vi "Helper - overlay optimal heading.vi"(6 "Line length (px)":dbl=500.0, 8 "Overlay Color":u32(colorbox)=6618880, 9 "Boat Image Coords":cluster{"X":i32, "Y":i32}, 10 "Optimal Heading":T2 format="%05.1f", 11 "Image In":T1) -> (3 "Image Out":T1)   [LabVIEW 2011]
doc: "overlays a line indicating the direction that the boat 'wants' to go.\nby Jason Curtis"
uses:
  <vilib>/vision/Image Controls.llb/IMAQ Image.ctl
  2-Think/2 Typedefs/heading.ctl
panel:
  out "Start Point":cluster{"X":i32, "Y":i32}
  out "End Point":cluster{"X":i32, "Y":i32}
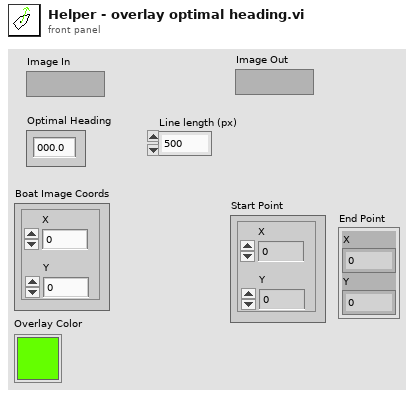
[diagram p1: front panel]
types:
  T1 = typedef "IMAQ Image.ctl" = refnum<image>
  T2 = typedef "heading.ctl" = dbl
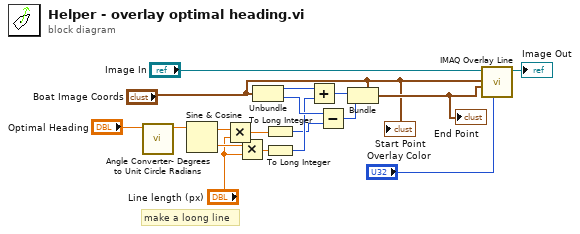
[diagram p0: block diagram]
diagram:
  # "make a loong line"
  n1 = call "Angle Converter- Degrees to Unit Circle Radians.vi"("Angle in \nHeading \nFormat"="Optimal Heading") -> ("Angle in \nUnit Circle\nRadians"=w16:dbl)  [unwired: 10 in]
  n2 = Sine & Cosine(0:w16) -> (1:w14:dbl, 2:w15:dbl)
  n3 = Multiply(x=w14, y="Line length (px)") -> (x*y=w8:dbl)
  n4 = Multiply(x=w15, y="Line length (px)") -> (x*y=w7:dbl)
  n5 = Unbundle("Boat Image Coords") -> ("X"=w12:i32, "Y"=w9:i32)
  n6 = To Long Integer(number=w8) -> (32bit integer=w4:i32)
  n7 = To Long Integer(number=w7) -> (32bit integer=w5:i32)
  n8 = Add(x=w12, y=w5) -> (x+y=w11:i32)
  n9 = Subtract(x=w9, y=w4) -> (x-y=w10:i32)
  n10 = Bundle(cluster="Boat Image Coords", "X"=w11, "Y"=w10) -> (w3:cluster{"X":i32, "Y":i32})
  "End Point" <- w3
  n11 = call "IMAQ Overlay Line"("Color"="Overlay Color", "End Point"=w3, "Start Point"="Boat Image Coords", "Image"="Image In") -> ("Image Out"=→"Image Out":T1)  [unwired: 6 in, 1 out]
  "Start Point" <- "Boat Image Coords"
